vi "Simulate Signal with Probe.vi"() -> ()   [LabVIEW 2021]
panel:
  in  "Frequency":dbl(knob) scale=0.0..10.0
  in  "Amplitude":dbl(knob) scale=0.0..10.0
  in  "stop":bool
  out "Waveform Chart":dynamicdata(graph)
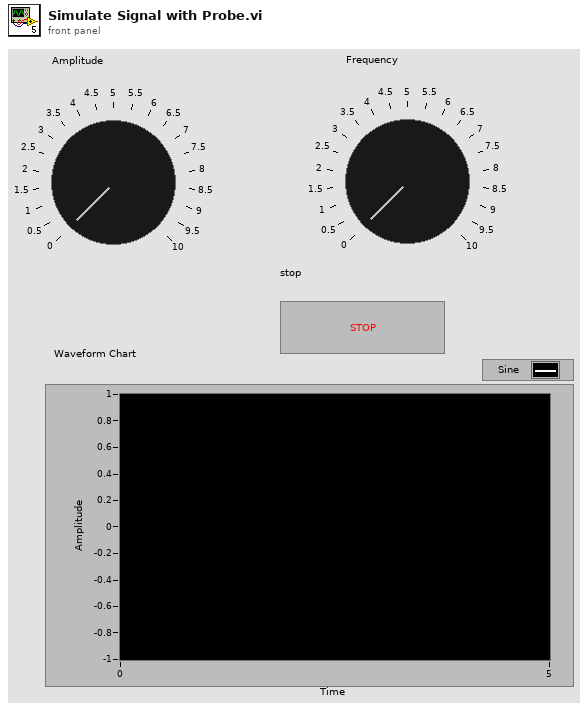
[diagram p1: front panel]
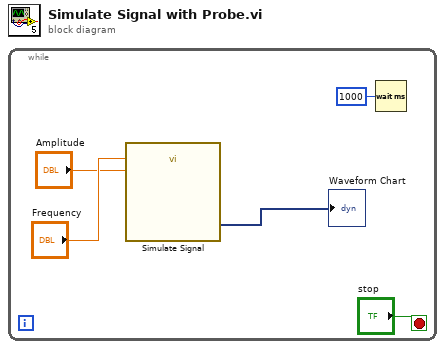
[diagram p0: block diagram]
diagram:
  n1 = while {
    stop <- "stop" stop-if-true
    n2 = call "Simulate Signal"("Frequency"="Frequency", "Amplitude"="Amplitude") -> ("Sine"=→"Waveform Chart":dynamicdata)  [unwired: 12 in, 1 out]
    n3 = Wait (ms)(milliseconds to wait=u32 1000) -> ()  [unwired: 1 out]
  }
